vi "Verify new image.vi"(8 "error in (no error)":errorcluster, 11 "CCDCamera in":refnum<class "Simulated Camera.lvclass">) -> (0 "error out":errorcluster, 2 "New Images ?":bool, 3 "CCDCamera out":refnum<class "Simulated Camera.lvclass">)   [LabVIEW 2018, in "Simulated Camera.lvclass"]
doc: "Verify is there is any new image"
uses:
  Simulated Camera.lvclass
  Simulated Camera.lvclass/Simulated Camera.ctl
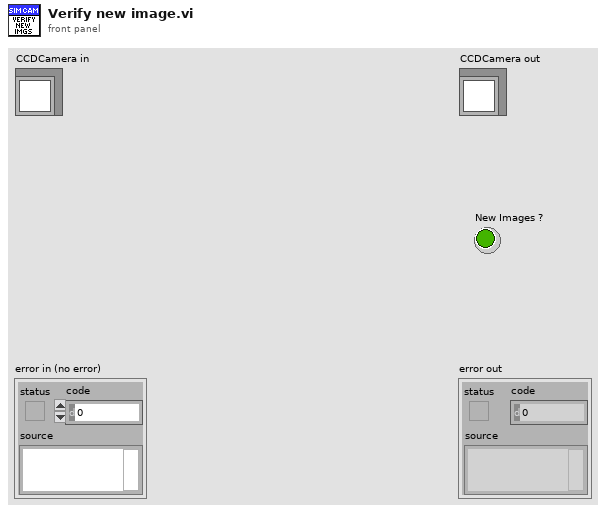
[diagram p1: front panel]
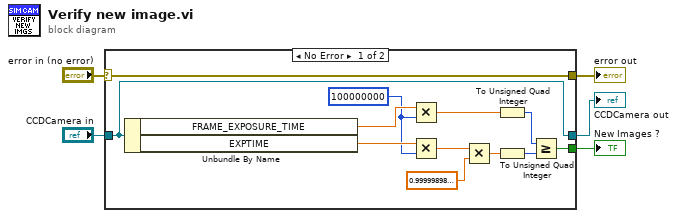
[diagram p0: block diagram]
diagram:
  n1 = case shown="No Error" "error in (no error)" {
    selector: "error in (no error)" -> [w17 w19]
    tunnel: [w17 w19] -> w4
    tunnel: [w16 w18] -> w2
    tunnel: "CCDCamera in" -> [w16 w18]
    tunnel: [w15 _] -> w1
    frame No Error {
      w12 = 100000000
      n2 = Unbundle By Name(w16) -> ("FRAME_EXPOSURE_TIME"=w14:sgl, "EXPTIME"=w13:dbl)
      n3 = Multiply(x=w14, y=w12) -> (x*y=w11:sgl)
      n4 = Multiply(x=w13, y=w12) -> (x*y=w7:dbl)
      n5 = Multiply(x=w7, y=sgl 0.999999) -> (x*y=w8:dbl)
      n6 = To Unsigned Quad Integer(1:w11) -> (0:w10:u64)
      n7 = To Unsigned Quad Integer(1:w8) -> (0:w6:u64)
      n8 = Greater Or Equal?(x=w10, y=w6) -> (x >= y?=w15:bool)
    }
    frame Error {
    }
  }
  "error out" <- w4
  "CCDCamera out" <- w2
  "New Images ?" <- w1
